vi "XY Chart Buffer.vi"(8 "clear first (no:F)":bool, 9 "chart length (points)":i32=100, 10 "new point":cluster{"x":dbl, "y":dbl} {"y" format="%.2f"; "x" format="%.2f"}, 11 "new points":cluster{"x":dbl, "y":dbl}[](array[cluster]) {"y" format="%.2f"; "x" format="%.2f"}) -> (3 "XY chart data":cluster{"x":dbl, "y":dbl}[](array[cluster]) {"y" format="%.2f"; "x" format="%.2f"})   [LabVIEW 2010]
doc: "This reentrant VI uses an XY graph to mimic the behavior of an XY chart, in that it plots a stipulated amount of the most recently acquired data points. The chart data is stored in a static local variable of the output XY chart indicator.\n\nBecause the VI has been marked reentrant (in VI setup), you can make multiple parallel calls to the VI without confusing the memory. Use the new points array input to supply multiple points at once, or leave the array unwired (empty) and use the new point cluster input to supply one point at a time. If the locally stored chart array is not equal to chart length, it is expanded to that lenght by replicating the most recently acquired point. Data in excess of the history length is discarded. Set clear first to clear the chart history before processing the new points."
panel:
  in  "Case Constant\n(See Context Help)":bool=TRUE
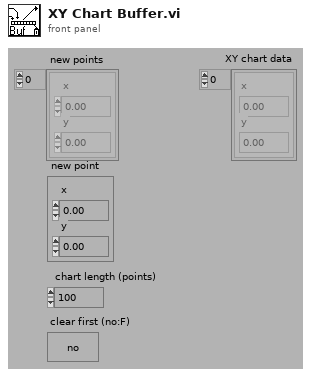
[diagram p1: front panel]
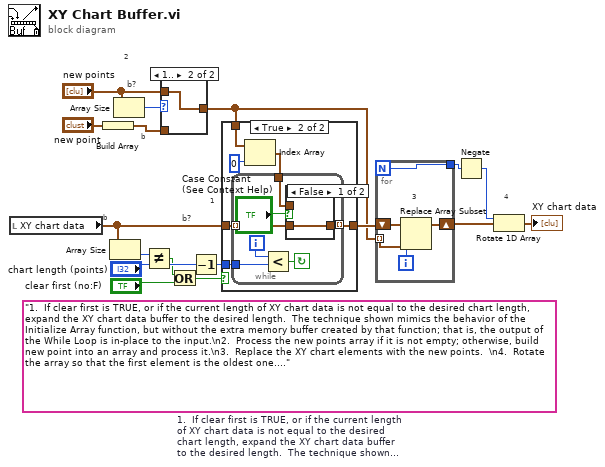
[diagram p0: block diagram]
diagram:
  (unwired) "1.  If clear first is TRUE, or if the current length of XY chart data is not equal to the desired chart length, expand the XY chart data buffer to the desired length.  The technique shown mimics the behavior of the Initialize Array function, but without the extra memory buffer created by that function; that is, the output of the While Loop is in-place to the input.\n2.  Process the new points array if it is not empty; otherwise, build new point into an array and process it.\n3.  Replace the XY chart elements with the new points.  \n4.  Rotate the array so that the first element is the oldest one.\nb marks a diagram array buffer; b? marks a buffer that may be in the calling VI. "  # 1.  If clear first is TRUE, or if the current length of XY chart data is not equal to the desired chart length, expand the XY chart data buffer to the desired length.  The technique shown mimics the behavior of the Initialize Array function, but without the extra memory buffer created by that function; that is, the output of the While Loop is in-place to the input. 2.  Process the new points array if it is not empty; otherwise, build new point into an array and process it. 3.  Replace the XY chart elements with the new points.   4.  Rotate the array so that the first element is the oldest one. b marks a diagram array buffer; b? marks a buffer that may be in the calling VI.
  # "b"
  # "4"
  # "2"
  # "1"
  # "b?"
  # "b"
  # "b?"
  n1 = local read "XY chart data"() -> (w2:cluster{"x":dbl, "y":dbl}[])
  n2 = Build Array("new point") -> (w17:cluster{"x":dbl, "y":dbl}[])
  n3 = Array Size(array=w2) -> (size(s)=w9:i32)
  n4 = Array Size(array="new points") -> (size(s)=w15:i32)
  n5 = Not Equal?(x=w9, y="chart length (points)") -> (x != y?=w6:bool)
  n6 = case shown="1.." w15 {
    tunnel: [w18 w19] -> w1
    tunnel: "new points" -> [_ w19]
    tunnel: w17 -> [w18 _]
    frame ..0 {
    }
    frame 1.. {
    }
  }
  n7 = Or(x=w6, y="clear first (no:F)") -> (x .or. y?=w5:bool)
  n8 = Decrement(x="chart length (points)") -> (x-1=w4:i32)
  n9 = case shown="True" w5 {
    tunnel: [w20 w21] -> w10
    tunnel: w4 -> [_ w25]
    tunnel: w2 -> [w20 w26]
    tunnel: w1 -> [_ w23]
    frame False {
    }
    frame True {
      n10 = Index Array(array=w23, index=0) -> (element=w22:cluster{"x":dbl, "y":dbl})
      n11 = while {
        tunnel: [w29] -> w21 mode=indexing
        tunnel: w22 -> [w27]
        tunnel: w25 -> [w33]
        tunnel: w26 -> [w28] mode=indexing
        i -> [w32]
        stop <- w31 continue-if-true
        n12 = Less?(x=w32, y=w33) -> (x < y?=w31:bool)
        n13 = case shown="False" "Case Constant\n(See Context Help)" {
          tunnel: [w34 w35] -> w29
          tunnel: w28 -> [w34 _]
          tunnel: w27 -> [_ w35]
          frame False {
          }
          frame True {
          }
        }
      }
    }
  }
  n14 = for {
    N -> [w36]
    shift-right: [w40] -> w12
    shift-left: w10 -> [w37]
    tunnel: w1 -> [w38] mode=indexing
    tunnel: [w36] -> w8
    i -> [w39]
    # "3"
    n15 = Replace Array Subset(array=w37, new element=w38, index=w39) -> (w40:cluster{"x":dbl, "y":dbl}[])
  }
  n16 = Negate(x=w8) -> (-x=w13:i32)
  n17 = Rotate 1D Array(1:w12, 2:w13) -> (0:→"XY chart data":cluster{"x":dbl, "y":dbl}[])
